vi "对中 偏差角度.vi"(9 "角度":dbl[](array[numeric]), 10 "油压":dbl[](array[numeric]), 11 "扭矩":dbl[](array[numeric])) -> (1 "偏差角度":dbl, 3 "偏差扭矩":dbl format="%0.2f")   [LabVIEW 2015, in "Logging.lvlib"]
uses:
  Logging.lvlib
  <vilib>/Analysis/1siggen.llb/Ramp Pattern by Samples.vi
  <vilib>/Analysis/baseanly.llb/Mean (DBL).vi
  <vilib>/gmath/NI_Gmath.lvlib
  <vilib>/Analysis/NI_AALBase.lvlib
panel:
  out "角度反转回":dbl[](array[numeric])
  out "角度反转去":dbl[](array[numeric])
  out "角度正转回":dbl[](array[numeric])
  out "角度正转去":dbl[](array[numeric])
  out "油压反转回":dbl[](array[numeric])
  out "油压反转去":dbl[](array[numeric])
  out "油压正转回":dbl[](array[numeric])
  out "油压正转去":dbl[](array[numeric])
  out "扭矩反转回":dbl[](array[numeric])
  out "扭矩反转去":dbl[](array[numeric])
  out "扭矩正转回":dbl[](array[numeric])
  out "扭矩正转去":dbl[](array[numeric])
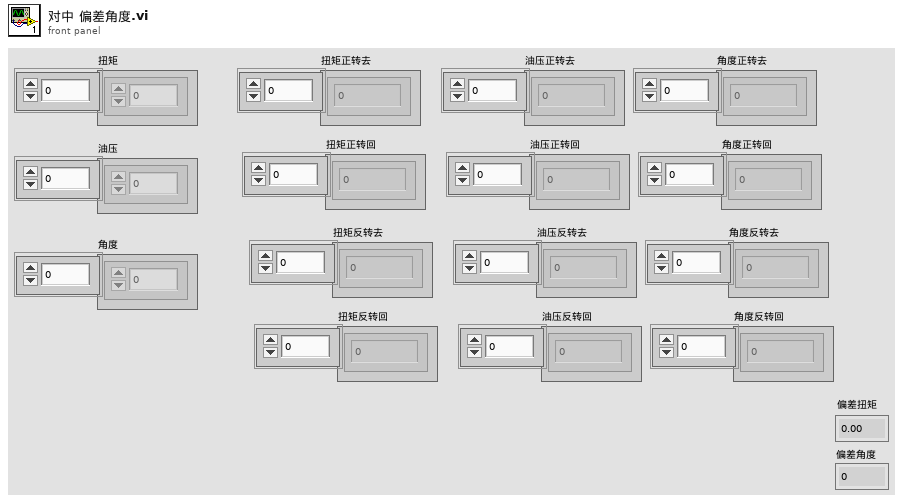
[diagram p1: front panel]
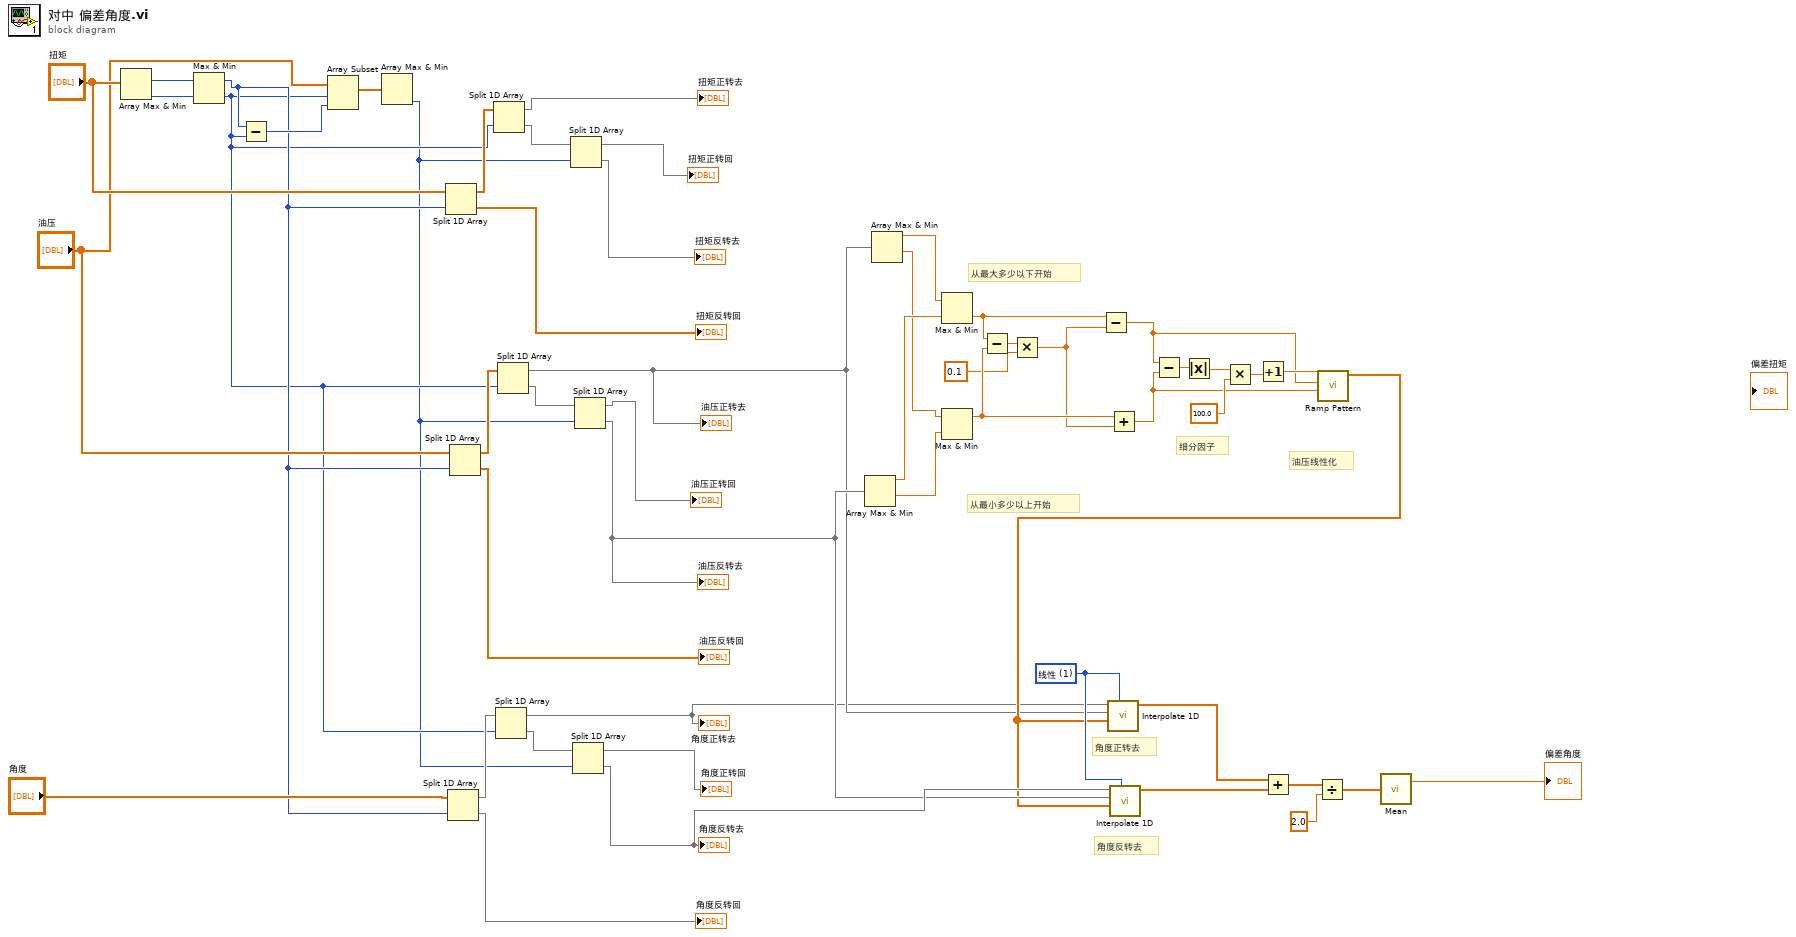
[diagram p0: block diagram]
diagram:
  w12 = 1 items=["最近", "线性", "样条", "cubic Hermite", "拉格朗日"] ("method")
  # "角度反转去"
  # "角度正转去"
  # "油压线性化"
  # "细分因子"
  # "从最大多少以下开始"
  # "从最小多少以上开始"
  n1 = Array Max & Min(array="扭矩") -> (max index (indices)=w52:i32, min index (indices)=w51:i32)  [unwired: 2 out]
  n2 = Max & Min(x=w52, y=w51) -> (max(x,y)=w38:i32, min(x,y)=w37:i32)
  n3 = Subtract(x=w38, y=w37) -> (x-y=w48:i32)
  n4 = Array Subset(array="油压", index=w37, length=w48) -> (w47:dbl[])
  n5 = Array Max & Min(array=w47) -> (min index (indices)=w36:i32)  [unwired: 3 out]
  n6 = Split 1D Array(array="扭矩", index=w38) -> (first subarray=w49:dbl[], second subarray=→"扭矩反转回":dbl[])
  n7 = Split 1D Array(array="角度", index=w38) -> (first subarray=w40:dbl[], second subarray=→"角度反转回":dbl[])
  n8 = Split 1D Array(array="油压", index=w38) -> (first subarray=w45:dbl[], second subarray=→"油压反转回":dbl[])
  n9 = Split 1D Array(array=w49, index=w37) -> (first subarray=→"扭矩正转去":dbl[], second subarray=w21:dbl[])
  n10 = Split 1D Array(array=w40, index=w37) -> (first subarray=w1:dbl[], second subarray=w20:dbl[])
  "角度正转去" <- w1
  n11 = Split 1D Array(array=w45, index=w37) -> (first subarray=w2:dbl[], second subarray=w44:dbl[])
  "油压正转去" <- w2
  n12 = Split 1D Array(array=w21, index=w36) -> (first subarray=→"扭矩正转回":dbl[], second subarray=→"扭矩反转去":dbl[])
  n13 = Split 1D Array(array=w20, index=w36) -> (first subarray=→"角度正转回":dbl[], second subarray=w11:dbl[])
  "角度反转去" <- w11
  n14 = Split 1D Array(array=w44, index=w36) -> (first subarray=→"油压正转回":dbl[], second subarray=w10:dbl[])
  "油压反转去" <- w10
  n15 = Array Max & Min(array=w10) -> (max value=w34:dbl, min value=w32:dbl)  [unwired: 2 out]
  n16 = Array Max & Min(array=w2) -> (max value=w35:dbl, min value=w33:dbl)  [unwired: 2 out]
  n17 = Max & Min(x=w35, y=w34) -> (min(x,y)=w18:dbl)  [unwired: 1 out]
  n18 = Max & Min(x=w33, y=w32) -> (max(x,y)=w17:dbl)  [unwired: 1 out]
  n19 = Subtract(x=w18, y=w17) -> (x-y=w16:dbl)
  n20 = Multiply(x=w16, y=0.1) -> (x*y=w14:dbl)
  n21 = Subtract(x=w18, y=w14) -> (x-y=w13:dbl)
  n22 = Add(x=w17, y=w14) -> (x+y=w26:dbl)
  n23 = Subtract(x=w13, y=w26) -> (x-y=w31:dbl)
  n24 = Absolute Value(x=w31) -> (abs(x)=w29:dbl)
  n25 = Multiply(x=w29, y=100.0) -> (x*y=w30:dbl)
  n26 = Increment(x=w30) -> (x+1=w27:dbl)
  n27 = call-poly <vilib>:"Ramp Pattern.vi"("start"=w26, "end"=w13, "samples"=w27) -> ("Ramp Pattern"=w9:dbl[])  [unwired: 7 in, 1 out]
  n28 = call <vilib>:"Interpolate 1D.vi"("method"=w12, "xi"=w9, "X"=w2, "Y"=w1) -> ("yi"=w8:dbl[])  [unwired: 5 in, 2 out]
  n29 = call <vilib>:"Interpolate 1D.vi"("method"=w12, "xi"=w9, "X"=w10, "Y"=w11) -> ("yi"=w7:dbl[])  [unwired: 5 in, 2 out]
  n30 = Add(x=w8, y=w7) -> (x+y=w6:dbl[])
  n31 = Divide(x=w6, y=2.0) -> (x/y=w4:dbl[])
  n32 = call-poly <vilib>:"Mean.vi"("X"=w4) -> ("mean"=→"偏差角度":dbl)  [unwired: 1 out]
